vi "target - multi rate.vi"() -> ()   [LabVIEW 2016]
uses:
  <vilib>/Platform/TimedLoop/XDataNode/timing_clust.ctl
  <vilib>/Platform/TimedLoop/XDataNode/nitl_modes.ctl
  <vilib>/Platform/TimedLoop/XDataNode/wakeup.ctl
  <vilib>/FPGAPlugInAG/cRIO-9066/niLvFpga_Open_cRIO-9066.vi
  <vilib>/rvi/interface/common/dynamic/niFpgaDynamicAddResources.vi
  <vilib>/FPGAPlugInAG/Dynamic/niLvFpga_Run_Dynamic.vi
  <vilib>/Utility/error.llb/Error Cluster From Error Code.vi
  <vilib>/rvi/errors/niLvFpgaAdjustHostInterfaceError.vi
  <vilib>/FPGAPlugInAG/Dynamic/niLvFpga_Close_Dynamic.vi
  <vilib>/rvi/interface/nirviOpenFPGA/nirviOpenFPGA.xnode
  FPGA Bitfiles/resFreq_FPGATarget_FPGAOutput_rADQ7i9uYWk.lvbitx
  <vilib>/rvi/interface/nirviMethod/nirviMethod.xnode
  <vilib>/Platform/TimedLoop/XDataNode/XDataNode.xnode
  <vilib>/rvi/interface/nirviReadWriteControl/nirviReadWriteControl.xnode
  <vilib>/rvi/interface/nirviCloseFPGA/nirviCloseFPGA.xnode
  NiFpgaLv.dll
  <vilib>/rvi/interface/Simulation/niFpgaSimulationCallBeginRW.vi
  <vilib>/Platform/TimedLoop/XDataNode/XDNodeRunTimeDep.lvlib
panel:
  in  "Both":bool caption="ON"
  in  "Ch1":bool caption="ON"
  in  "Ch0":bool caption="ON"
  in  "Amplitude [V]":dbl
  in  "Frequency [Hz]":dbl
  in  "stop":bool
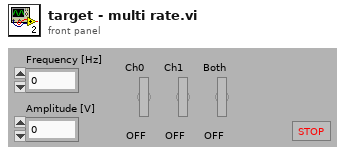
[diagram p1: front panel]
types:
  T1 = typedef "XDNodeRunTimeDep.lvlib/timing_clust.ctl" = cluster{"Expected End [f-1]":u64, "Actual End [f-1]":u64, "Finished Late? [f-1]":bool, "Expected End [i-1]":u64, "Actual End [i-1]":u64, "Finished Late? [i-1]":bool, "Expected Start [i]":u64, "Actual Start [i]":u64, "Expected Start [f]":u64, "Actual Start [f]":u64, "Source Name":string, "Structure Name":string, "Period":i64, "Deadline":i64, "Offset":i64, "Start":i64, "Priority":i32, "Timeout":i32, "Mode":T2, "Wakeup Reason":T3, "Error":errorcluster, "Source Type":string, "Secondary Source Type":string, "Global End Time":u64, "Global Start Time":u64, "Frame Duration":u64, "Iteration Duration":u64, "Assigned CPU":i32, "I/O Scan Engine Mode":u32}
  T2 = typedef "XDNodeRunTimeDep.lvlib/nitl_modes.ctl" = enum32{"No Change", "Process missed periods, maintain original phase", "Discard missed periods, maintain original phase", "Process missed periods, ignore original phase", "Discard missed periods, ignore original phase"}
  T3 = typedef "XDNodeRunTimeDep.lvlib/wakeup.ctl" = enum32{"Normal", "Aborted", "Asynchronous wakeup", "Timing source error", "Timed loop error", "Timeout"}
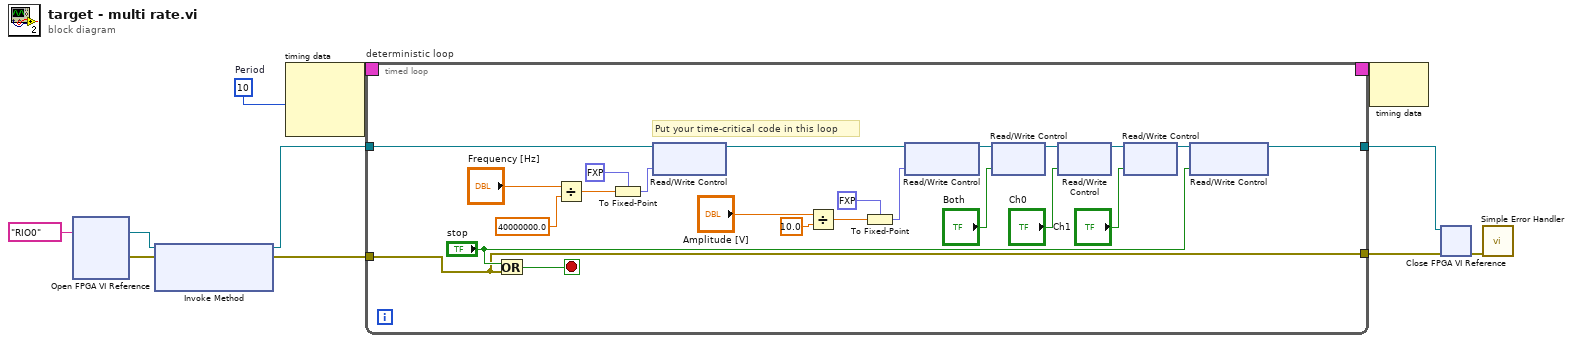
[diagram p0: block diagram]
diagram:
  w4 = i64 10  # Period
  n1 = xnode "Open FPGA VI Reference"("resource name"=tag "RIO0") -> ("FPGA VI Reference Out"=w8:refnum<k20>, "error out"=w9:errorcluster)  [unwired: 1 in]
  n2 = xnode "Invoke Method"("FPGA VI Reference In"=w8, "error in"=w9) -> ("FPGA VI Reference Out"=w11:refnum<k20>, "error out"=w3:errorcluster)  [unwired: 1 in]
  n3 = node-c288 ("Input Node")(w4) -> (w6:T1)  [unwired: 2 in]
  n4 = timed-loop "deterministic loop" {
    timing: w6 -> [_]
    timing-out: [_] -> w5
    tunnel: [w34] -> w1
    tunnel: [w20] -> w2
    tunnel: w3 -> [w20]
    tunnel: w11 -> [w19]
    stop <- w33 stop-if-true
    # "Put your time-critical code in this loop"
    n5 = Or(x="stop", y=w20) -> (x .or. y?=w33:bool)
    n6 = Divide(x="Frequency [Hz]", y=40000000.0) -> (x/y=w26:dbl)
    n7 = To Fixed-Point(fixed-point type=fxp<+,32,0> 0.0 ("frequency (periods/tick)"), number=w26) -> (fixed-point=w25:fxp<+,32,0>)
    n8 = xnode "Read/Write Control"("FPGA VI Reference In"=w19, "Frequency"=w25) -> ("FPGA VI Reference Out"=w32:refnum<k20>)  [unwired: 1 in, 1 out]
    n9 = Divide(x="Amplitude [V]", y=10.0) -> (x/y=w23:dbl)
    n10 = To Fixed-Point(fixed-point type=fxp<+,32,0> 0.0 ("Amplitude"), number=w23) -> (fixed-point=w24:fxp<+,32,0>)
    n11 = xnode "Read/Write Control"("FPGA VI Reference In"=w32, "Amplitude"=w24) -> ("FPGA VI Reference Out"=w18:refnum<k20>)  [unwired: 1 in, 1 out]
    n12 = xnode "Read/Write Control"("FPGA VI Reference In"=w18, "Both"="Both") -> ("FPGA VI Reference Out"=w17:refnum<k20>)  [unwired: 1 in, 1 out]
    n13 = xnode "Read/Write Control"("FPGA VI Reference In"=w17, "Ch0"="Ch0") -> ("FPGA VI Reference Out"=w16:refnum<k20>)  [unwired: 1 in, 1 out]
    n14 = xnode "Read/Write Control"("FPGA VI Reference In"=w16, "Ch1"="Ch1") -> ("FPGA VI Reference Out"=w15:refnum<k20>)  [unwired: 1 in, 1 out]
    n15 = xnode "Read/Write Control"("FPGA VI Reference In"=w15, "StopButton"="stop") -> ("FPGA VI Reference Out"=w34:refnum<k20>)  [unwired: 1 in, 1 out]
  }
  n16 = node-c288 ("Output Node")(w5) -> ()  [unwired: 1 out]
  n17 = xnode "Close FPGA VI Reference"("FPGA VI Reference In"=w1, "error in"=w2) -> ("error out"=w10:errorcluster)
  n18 = call <vilib>:"Simple Error Handler.vi"("error in (no error)"=w10) -> ()  [unwired: 4 in, 5 out]
